vi "upq.vi"(9 "ImagenBinaria":u32[][](array[numeric]), 10 "q":dbl=1.0 format="%#_13g", 11 "p":dbl=1.0 format="%#_13g") -> (3 "upq":dbl)   [LabVIEW 2021]
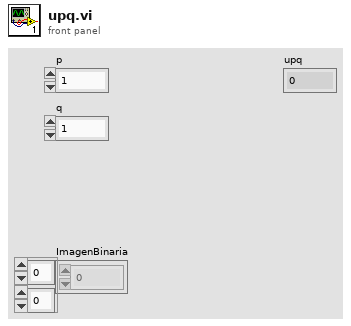
[diagram p1: front panel]
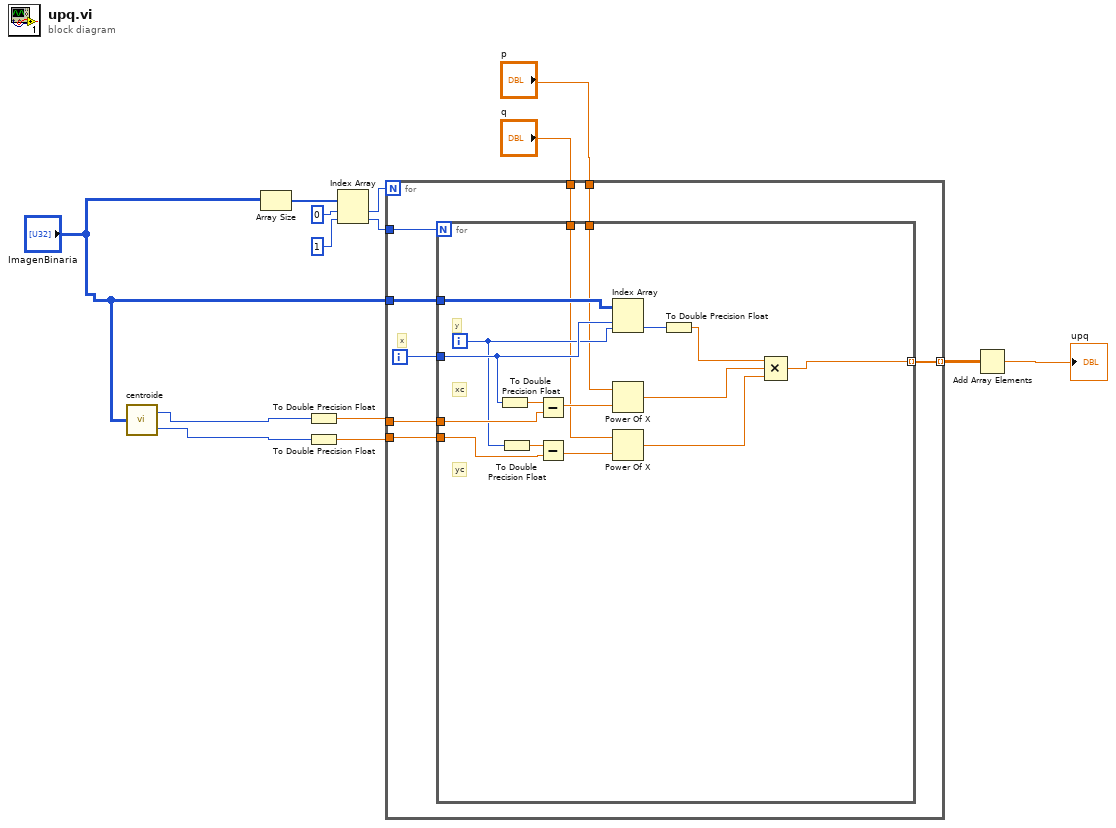
[diagram p0: block diagram]
diagram:
  n1 = call "centroide.vi"("Array 2"="ImagenBinaria") -> ("cx"=w3:u16, "cy"=w2:u16)
  n2 = Array Size(array="ImagenBinaria") -> (size(s)=w4:i32[])
  n3 = To Double Precision Float(number=w3) -> (double precision float=w9:dbl)
  n4 = To Double Precision Float(number=w2) -> (double precision float=w10:dbl)
  n5 = Index Array(array=w4, index #1=0 ("index"), index #2=1 ("index")) -> (element #1=w7:i32, element #2=w8:i32)
  n6 = for {
    N: w7 -> [_]
    tunnel: w8 -> [w22]
    tunnel: "ImagenBinaria" -> [w21]
    tunnel: w9 -> [w19]
    tunnel: w10 -> [w18]
    tunnel: [w17] -> w11 mode=indexing
    tunnel: "p" -> [w16]
    tunnel: "q" -> [w15]
    i -> [w20]
    # "x"
    n7 = for {
      N: w22 -> [_]
      tunnel: w21 -> [w38]
      tunnel: w20 -> [w36]
      tunnel: w19 -> [w37]
      tunnel: w18 -> [w34]
      tunnel: [w28] -> w17 mode=indexing
      tunnel: w16 -> [w26]
      tunnel: w15 -> [w25]
      i -> [w35]
      # "y"
      # "yc"
      # "xc"
      n8 = To Double Precision Float(number=w36) -> (double precision float=w24:dbl)
      n9 = To Double Precision Float(number=w35) -> (double precision float=w23:dbl)
      n10 = Subtract(x=w24, y=w37) -> (x-y=w33:dbl)
      n11 = Subtract(x=w23, y=w34) -> (x-y=w32:dbl)
      n12 = Index Array(array=w38, index (row)=w36, index (col)=w35) -> (element=w27:u32)
      n13 = Power Of X(1:w33, 2:w26) -> (0:w31:dbl)
      n14 = Power Of X(1:w32, 2:w25) -> (0:w30:dbl)
      n15 = To Double Precision Float(number=w27) -> (double precision float=w29:dbl)
      n16 = Compound Arithmetic op=MULTIPLY(w29, w31, w30) -> (w28:dbl)
    }
  }
  n17 = Add Array Elements(numeric array=w11) -> (sum=→"upq":dbl)
